vi "Connect.vi"(8 "error in (no error)":errorcluster, 9 "Timeout (ms) (Default: 10s)":u32=10000, 10 "Receiver Timeout (ms) (Default: 50ms)":u32=50, 11 "COM Port":refnum<visa-resource-name>) -> (0 "error out":errorcluster, 3 "EPU452 out":refnum<class "EPU452.lvclass">)   [LabVIEW 2018, in "EPU452.lvclass"]
uses:
  EPU452.lvclass
  EPU452.lvclass/EPU452.ctl
  <vilib>/Instr/_visa.llb/VISA Configure Serial Port (Instr).vi
panel:
  in  "EPU452 in":refnum<class "EPU452.lvclass">
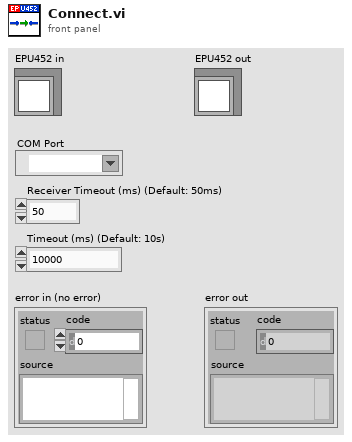
[diagram p1: front panel]
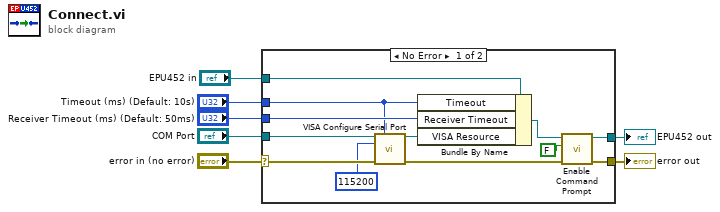
[diagram p0: block diagram]
diagram:
  n1 = case shown="No Error" "error in (no error)" {
    selector: "error in (no error)" -> [w17 w20]
    tunnel: "COM Port" -> [w19 _]
    tunnel: "EPU452 in" -> [w18 w21]
    tunnel: [w13 w20] -> w3
    tunnel: [w14 w21] -> w4
    tunnel: "Timeout (ms) (Default: 10s)" -> [w10 _]
    tunnel: "Receiver Timeout (ms) (Default: 50ms)" -> [w11 _]
    frame No Error {
      n2 = call-poly "VISA Configure Serial Port"("VISA resource name"=w19, "timeout (10sec)"=w10, "baud rate (9600)"=u32 115200, "error in (no error)"=w17) -> ("VISA resource name out"=w9:refnum<visa-resource-name>, "error out"=w8:errorcluster)  [unwired: 10 in]
      n3 = Bundle By Name(cluster=w18, "Timeout"=w10, "Receiver Timeout"=w11, "VISA Resource"=w9) -> (w15:refnum<class "EPU452.lvclass">)
      n4 = call "Enable Command Prompt.vi"("error in (no error)"=w8, "Enable Command Prompt?"=FALSE, "EPU452 in"=w15) -> ("error out"=w13:errorcluster, "EPU452 out"=w14:refnum<class "EPU452.lvclass">)  [unwired: 6 in, 1 out]
    }
    frame Error {
    }
  }
  "error out" <- w3
  "EPU452 out" <- w4
